vi "Convert to DarkSky API Time.vi"(8 "error in (no error)":errorcluster, 11 "Data/Time In":timestamp=timestamp(3584410380 s since 1904-01-01)) -> (0 "error out":errorcluster, 3 "DarkSky Time Out":dbl format="%#_10g")   [LabVIEW 2017, in "Dark Sky Weather Data for LabVIEW.lvlib"]
doc: "Use this VI to convert a LabVIEW Date/Time time stamp (UTC format) to the time value used by the DarkSky API (UNIX time)"
uses:
  Dark Sky Weather Data for LabVIEW.lvlib
  <vilib>/Utility/miscctls.llb/LVDateTimeRec.ctl
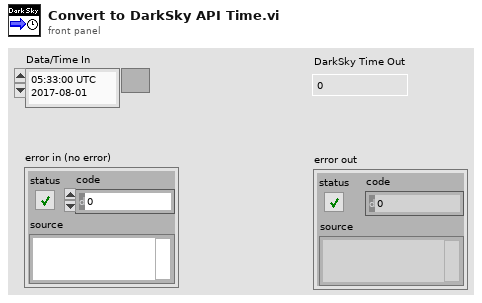
[diagram p1: front panel]
types:
  T1 = typedef "LVDateTimeRec.ctl" = cluster{"fractional second":dbl, "second":i32, "minute":i32, "hour":i32, "day of month":i32, "month":i32, "year":i32, "day of week":i32, "day of year":i32, "DST":i32}
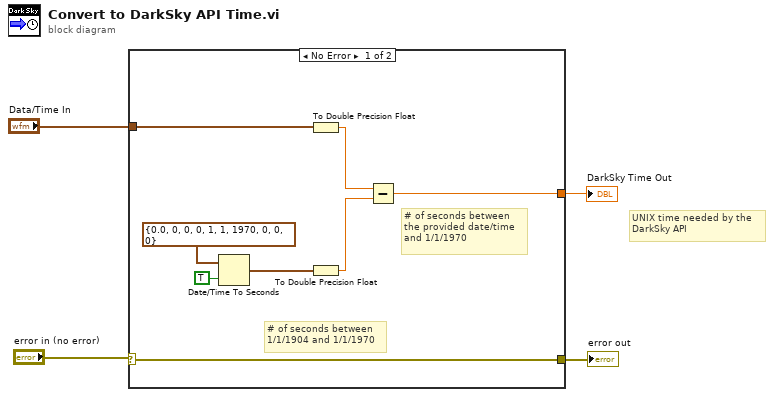
[diagram p0: block diagram]
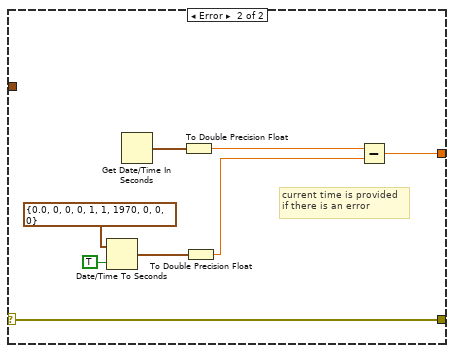
[diagram p2: hidden frame]
diagram:
  # "UNIX time needed by the\nDarkSky API"
  n1 = case shown="No Error" "error in (no error)" {
    selector: "error in (no error)" -> [w9 w20]
    tunnel: [w9 w20] -> w3
    tunnel: "Data/Time In" -> [w8 _]
    tunnel: [w5 w15] -> w1
    frame No Error {
      # "# of seconds between\nthe provided date/time\nand 1/1/1970"
      # "# of seconds between\n1/1/1904 and 1/1/1970"
      n2 = Date/Time To Seconds(1:TRUE ("is UTC (F)"), 2:T1 {"fractional second"=0.0, "second"=0, "minute"=0, "hour"=0, "day of month"=1, "month"=1, "year"=1970, "day of week"=0, "day of year"=0, "DST"=0} ("date time rec")) -> (0:w10:timestamp)
      n3 = To Double Precision Float(number=w8) -> (double precision float=w7:dbl)
      n4 = To Double Precision Float(number=w10) -> (double precision float=w6:dbl)
      n5 = Subtract(x=w7, y=w6) -> (x-y=w5:dbl)
    }
    frame Error {
      # "current time is provided\nif there is an error"
      n6 = Date/Time To Seconds(1:TRUE ("is UTC (F)"), 2:T1 {"fractional second"=0.0, "second"=0, "minute"=0, "hour"=0, "day of month"=1, "month"=1, "year"=1970, "day of week"=0, "day of year"=0, "DST"=0} ("date time rec")) -> (0:w16:timestamp)
      n7 = Get Date/Time In Seconds() -> (seconds since 1Jan1904=w19:timestamp)
      n8 = To Double Precision Float(number=w19) -> (double precision float=w14:dbl)
      n9 = To Double Precision Float(number=w16) -> (double precision float=w13:dbl)
      n10 = Subtract(x=w14, y=w13) -> (x-y=w15:dbl)
    }
  }
  "DarkSky Time Out" <- w1
  "error out" <- w3
